vi "Read Diode.vi"(8 "error in (no error)":errorcluster, 11 "Simulated DMM in":refnum<class "Simulated DMM.lvclass">) -> (0 "error out":errorcluster, 2 "Diode Voltage":dbl, 3 "Simulated DMM out":refnum<class "Simulated DMM.lvclass">)   [LabVIEW 2011, in "Simulated DMM.lvclass"]
uses:
  Simulated DMM.lvclass
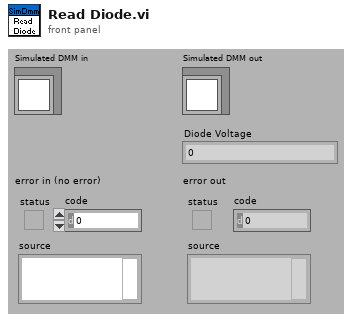
[diagram p1: front panel]
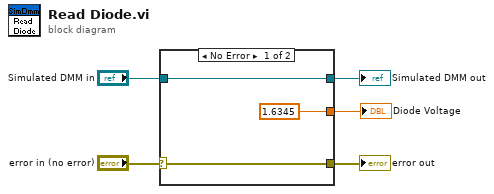
[diagram p0: block diagram]
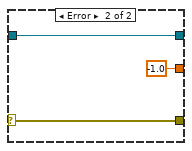
[diagram p2: hidden frame]
diagram:
  n1 = case shown="No Error" "error in (no error)" {
    selector: "error in (no error)" -> [w7 w10]
    tunnel: "Simulated DMM in" -> [w8 w11]
    tunnel: [w8 w11] -> w4
    tunnel: [w7 w10] -> w2
    tunnel: [1.6345 -1.0] -> w1
    frame No Error {
    }
    frame Error {
    }
  }
  "error out" <- w2
  "Simulated DMM out" <- w4
  "Diode Voltage" <- w1
